vi "Preprocessor.vi"() -> ()   [LabVIEW 2018]
uses:
  <vilib>/userdefined/High Color/IMAQdx.ctl
  <vilib>/vision/driver/IMAQdx.llb/IMAQdx Buffer Number Mode.ctl
  <vilib>/vision/driver/NI_Vision_Acquisition_Software.lvlib
  <vilib>/vision/NI_Vision_Development_Module.lvlib
panel:
  out "Processed 3":T1(plugin-control)
  out "MulFLAG":i32
  out "FLAG":i32
  out "FLAG":u8
  in  "Stop":bool
  in  "选项卡控件":T2(tab)
  in  "Method Select":T3(tab)
  in  "Start":bool
  in  "BINARY RANGE":cluster{u8, u8}(slide) scale=0.255..255.0
  out "Histogram":T4(graph)
  in  "Show Histo":bool
  in  "Equalize":bool
  in  "Process":bool
  in  "Operator":T5(ring)
  in  "X Val":sgl
  in  "RGBorGrey":bool
  in  "Range":cluster{"Numeric":sgl, "Numeric":sgl}(slide) scale=0.0..255.0
  in  "PackorCanny":bool
  in  "CANNY":bool
  in  "EDGE":bool
  in  "Edge Pack":T6(ring)
  in  "Canny Params":T7
  in  "Enable":bool
  in  "LOW               HIGH":bool
  in  "Frequency":bool
  in  "Plane":T8(ring)
  in  "Truncation Frequency %":sgl=10.0 format="%.2f"
  in  "Default or Personal":bool
  in  "Enable 2":bool
  out "Array":sgl[][](array[numeric])
  in  "Kernel Size":i32=3 min=3 max=7 step=2
  in  "Method":T9(ring)
  in  "Enable 3":bool
  in  "Kernel":string
  in  "Select":u16(ring) items=["Processed", "Origin"]
  in  "Camera Setting":T10
  out "Origin":T1(plugin-control)
  out "Processed":T1(plugin-control)
  in  "Save Image":bool
  in  "File Path":path
  in  "File Name":string
  in  "Method Control":enum32{"Single Operation", "Multiple Operation"}(tab)
  in  "Grey Trans":bool
  in  "Blur":bool
  in  "Symmetry":bool
  in  "Shift":bool
  in  "Rotate":bool
  in  "Binary":bool
  in  "Grey Trans 2":bool
  in  "Enable":bool
  in  "Blur 2":bool
  in  "Symmetry 2":bool
  in  "Shift 2":bool
  in  "Rotate 2":bool
  in  "Binary 2":bool
  out "Loading...":i32(slide) scale=-1.0..16.0
  out "Output Data Directory Path":path
  in  "Choose File 2":bool
  in  "Image Name":string
  in  "Generate number":i32
  out "Source Data File Path":path
  in  "Image format":string(combo)
  in  "Choose File":bool
  out "Processed 2":T1(plugin-control)
  # "Display"
  # "- Processed -"
  # "- Origin -"
  # "Threshold Image Processing:\n\n1. Start to process.\n2. You can scale the bar to change the\nthreshold of the algorithm.\n3. Click the Save button to save the pr\nocessed image."
  # "Gray Transform:\n\n1. Click Start button.\n2. Change the operator.\n3. Equalize histogram.\n4. Click Save button to Save image."
  # "Grey"
  # "RGB"
  # "Edge Detection\n\n1. Click Detect button.\n2. Change the Edge Pack.\n3. You can also choose canny detector.\n4. Click Save button to Save image."
  # "Canny"
  # "Pack"
  # "Frequency Processing:\n\n1. Click To Frequency Domain button.\n2. Change the Plane, you'll see the fre-\nquency image after FFT and FFTshift.\n3. You can also filter image based on \nhigh pass filter or low pass filter.\n4. Click Save button to save processed\nimage."
  # "High pass and Low pass Filter"
  # "Frequency Processing:\n\n1. Choose Default Mode or Personal\nMode.\n2. Click Enable button.\n3. Save images if you want."
  # "Personal"
  # "Default"
  # "Source Data"
  # "- Image Preview -"
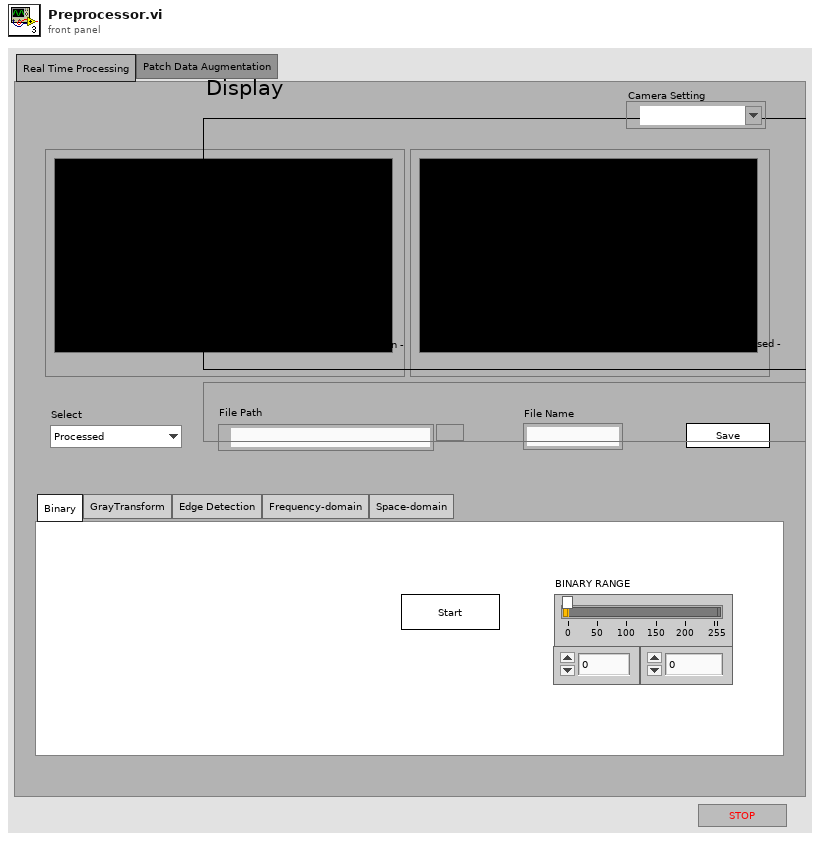
[diagram p1: front panel]
types:
  T1 = typedef "IMAQ Image.ctl" = refnum<image>
  T2 = enum32{"Real Time Processing", "Patch Data Augmentation"}
  T3 = enum32{"Binary", "GrayTransform", "Edge Detection", "Frequency-domain", "Space-domain"}
  T4 = cluster{"Starting Value":sgl, "Incremental Value":sgl, "Histogram":u32[]}
  T5 = enum32{"Linear", "Log", "Exp", "Square", "Square root", "Power X", "Power 1/X"}
  T6 = enum32{"Differentiation", "Gradient", "Prewitt", "Roberts", "Sigma", "Sobel"}
  T7 = cluster{"Sigma":sgl, "HThresh":sgl, "LThres":sgl, "WindowSize":i32}
  T8 = enum32{"Real", "Imaginary", "Magnitude", "Phase"}
  T9 = enum32{"", "Gradient", "Laplacian", "Smoothing", "Gaussian"}
  T10 = typedef "IMAQdx.ctl" = refnum<k21>
  T11 = typedef "Image Type" = u32
  T12 = typedef "NI_Vision_Acquisition_Software.lvlib/IMAQdx Buffer Number Mode.ctl" = enum32{"Next", "Last", "Buffer Number", "Every", "Last New"}
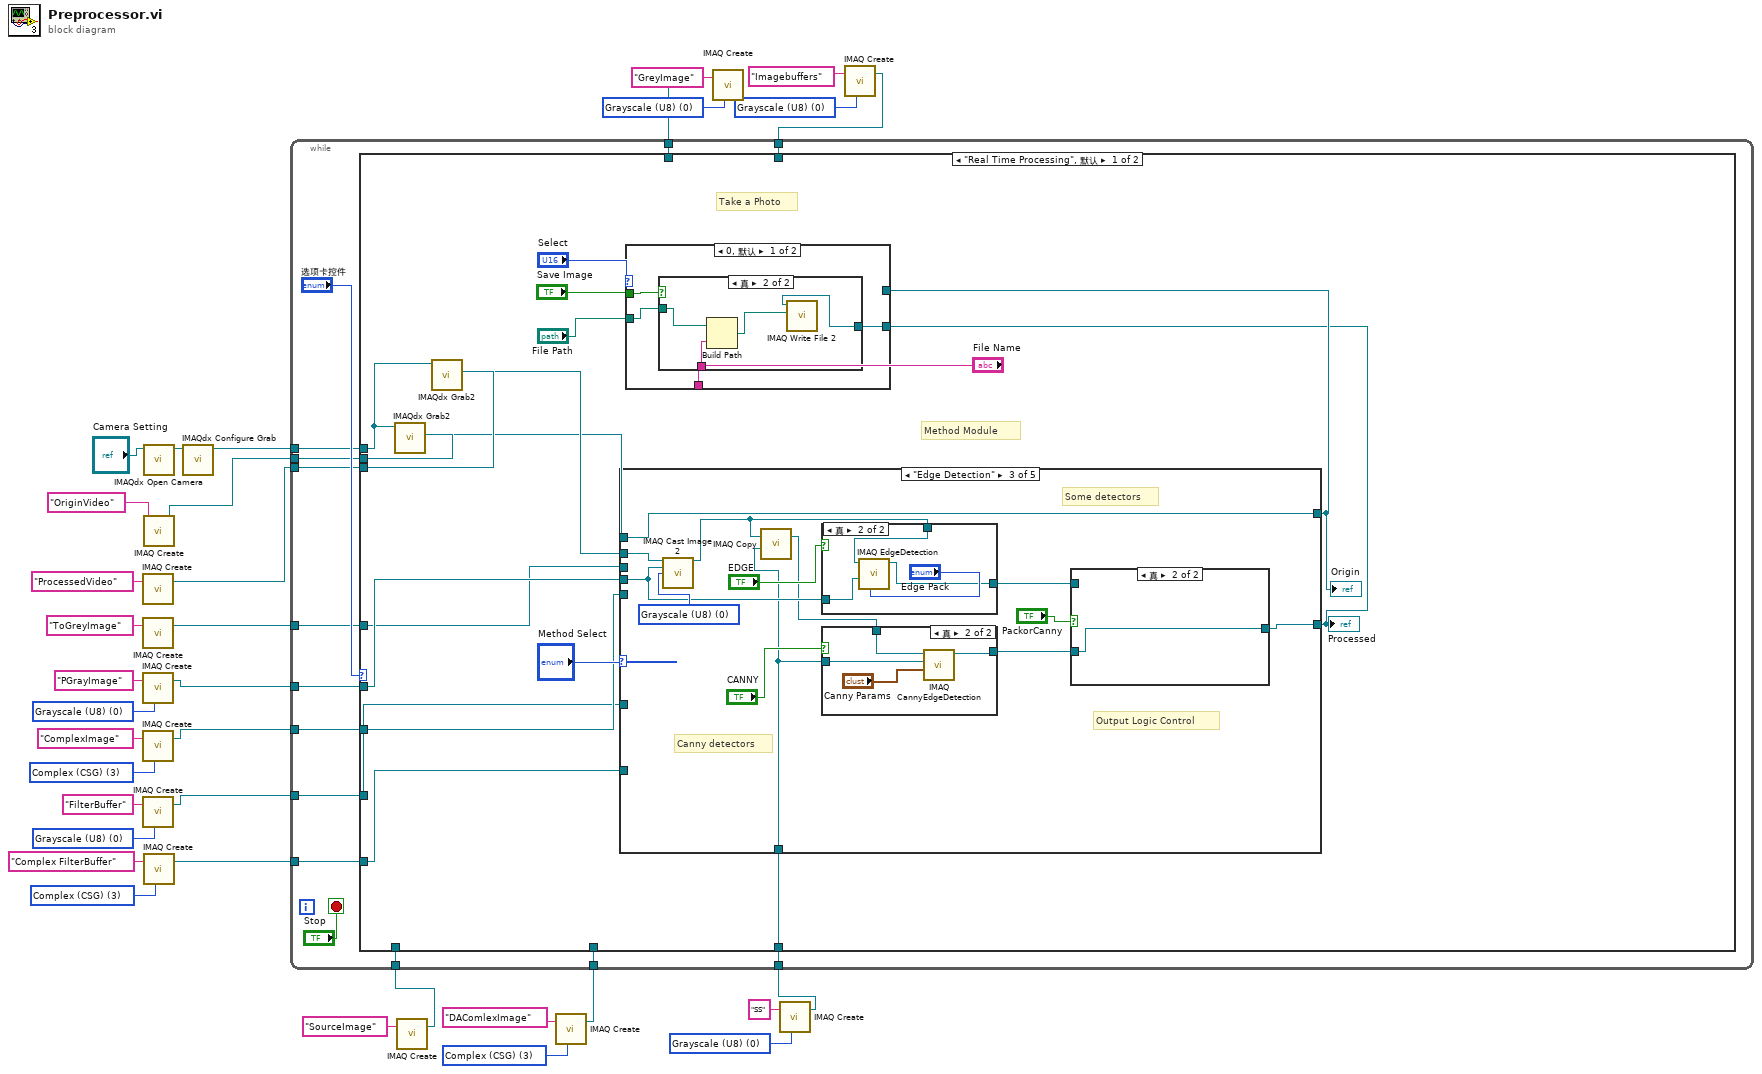
[diagram p0: block diagram]
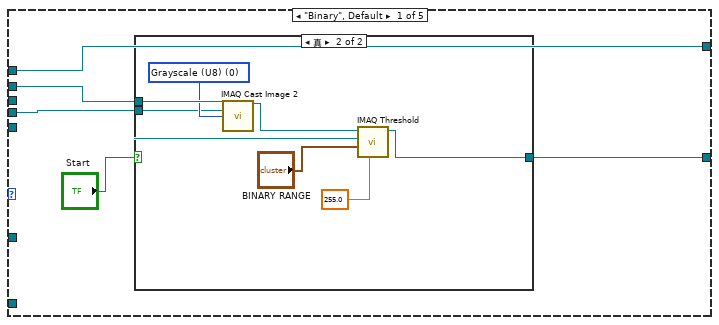
[diagram p2: hidden frame]
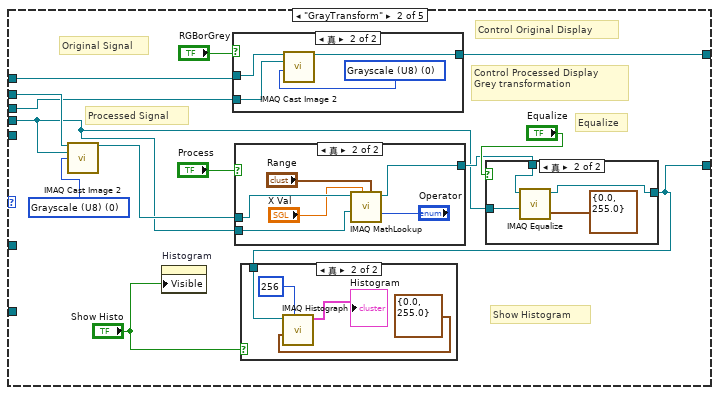
[diagram p4: hidden frame]
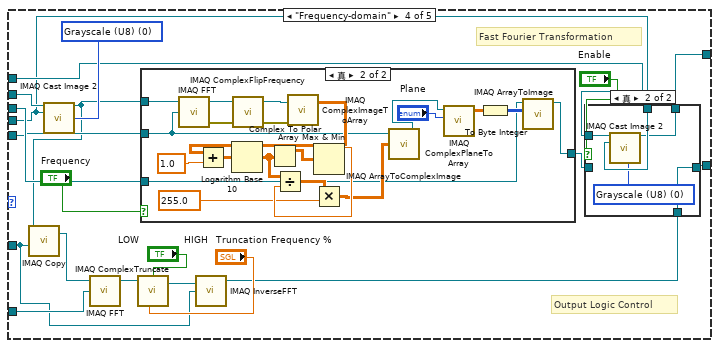
[diagram p12: hidden frame]
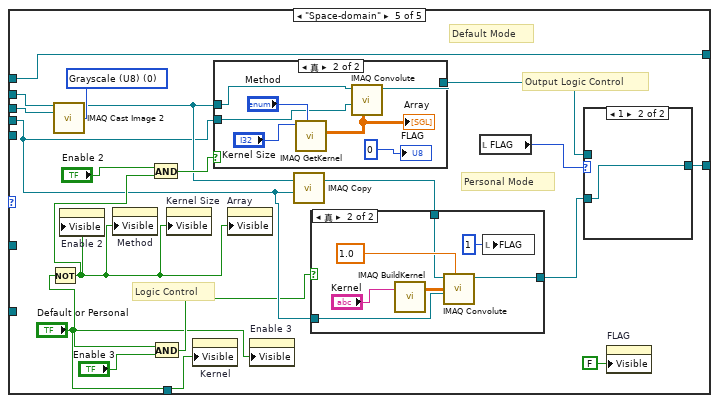
[diagram p15: hidden frame]
diagram:
  w3 = T11 0 items=["Grayscale (U8)", "Grayscale (I16)", "Grayscale (SGL)", "Complex (CSG)", "RGB (U32)", "HSL (U32)", "RGB (U64)", "Grayscale (U16)"] ("Image Type")
  w5 = T11 3 items=["Grayscale (U8)", "Grayscale (I16)", "Grayscale (SGL)", "Complex (CSG)", "RGB (U32)", "HSL (U32)", "RGB (U64)", "Grayscale (U16)"] ("Image Type")
  w8 = T11 0 items=["Grayscale (U8)", "Grayscale (I16)", "Grayscale (SGL)", "Complex (CSG)", "RGB (U32)", "HSL (U32)", "RGB (U64)", "Grayscale (U16)"] ("Image Type")
  w11 = T11 0 items=["Grayscale (U8)", "Grayscale (I16)", "Grayscale (SGL)", "Complex (CSG)", "RGB (U32)", "HSL (U32)", "RGB (U64)", "Grayscale (U16)"] ("Image Type")
  w16 = T11 3 items=["Grayscale (U8)", "Grayscale (I16)", "Grayscale (SGL)", "Complex (CSG)", "RGB (U32)", "HSL (U32)", "RGB (U64)", "Grayscale (U16)"] ("Image Type")
  w19 = T11 0 items=["Grayscale (U8)", "Grayscale (I16)", "Grayscale (SGL)", "Complex (CSG)", "RGB (U32)", "HSL (U32)", "RGB (U64)", "Grayscale (U16)"] ("Image Type")
  w22 = T11 3 items=["Grayscale (U8)", "Grayscale (I16)", "Grayscale (SGL)", "Complex (CSG)", "RGB (U32)", "HSL (U32)", "RGB (U64)", "Grayscale (U16)"] ("Image Type")
  w24 = T11 0 items=["Grayscale (U8)", "Grayscale (I16)", "Grayscale (SGL)", "Complex (CSG)", "RGB (U32)", "HSL (U32)", "RGB (U64)", "Grayscale (U16)"] ("Image Type")
  n1 = call "IMAQ Create"("Image Name"="ProcessedVideo") -> ("New Image"=w29:T1)  [unwired: 4 in, 1 out]
  n2 = call "IMAQ Create"("Image Name"="ToGreyImage") -> ("New Image"=w27:T1)  [unwired: 4 in, 1 out]
  n3 = call "IMAQ Create"("Image Name"="PGrayImage", "Image Type"=w24) -> ("New Image"=w25:T1)  [unwired: 3 in, 1 out]
  n4 = call "IMAQ Create"("Image Name"="ComplexImage", "Image Type"=w22) -> ("New Image"=w21:T1)  [unwired: 3 in, 1 out]
  n5 = call "IMAQ Create"("Image Name"="FilterBuffer", "Image Type"=w19) -> ("New Image"=w18:T1)  [unwired: 3 in, 1 out]
  n6 = call <vilib>:"IMAQdx Open Camera.vi"("Session In"="Camera Setting") -> ("Session Out"=w34:T10)  [unwired: 9 in, 1 out]
  n7 = call "IMAQ Create"("Image Name"="OriginVideo") -> ("New Image"=w31:T1)  [unwired: 4 in, 1 out]
  n8 = call "IMAQ Create"("Image Name"="Complex FilterBuffer", "Image Type"=w16) -> ("New Image"=w15:T1)  [unwired: 3 in, 1 out]
  n9 = call <vilib>:"IMAQdx Configure Grab.vi"("Session In"=w34) -> ("Session Out"=w32:T10)  [unwired: 9 in, 1 out]
  n10 = call "IMAQ Create"("Image Name"="SourceImage") -> ("New Image"=w13:T1)  [unwired: 4 in, 1 out]
  n11 = call "IMAQ Create"("Image Name"="DAComlexImage", "Image Type"=w5) -> ("New Image"=w4:T1)  [unwired: 3 in, 1 out]
  n12 = call "IMAQ Create"("Image Name"="GreyImage", "Image Type"=w11) -> ("New Image"=w10:T1)  [unwired: 3 in, 1 out]
  n13 = call "IMAQ Create"("Image Name"="SS", "Image Type"=w3) -> ("New Image"=w1:T1)  [unwired: 3 in, 1 out]
  n14 = call "IMAQ Create"("Image Name"="Imagebuffers", "Image Type"=w8) -> ("New Image"=w7:T1)  [unwired: 3 in, 1 out]
  n15 = while {
    tunnel: w32 -> [w48]
    tunnel: w31 -> [w47]
    tunnel: w29 -> [w46]
    tunnel: w27 -> [w45]
    tunnel: w25 -> [w44]
    tunnel: w21 -> [w43]
    tunnel: w18 -> [w42]
    tunnel: w15 -> [w41]
    tunnel: w13 -> [w40]
    tunnel: w10 -> [w39]
    tunnel: w7 -> [w38]
    tunnel: w4 -> [w37]
    tunnel: w1 -> [w36]
    stop <- "Stop" stop-if-true
    n16 = case shown="\"Real Time Processing\", 默认" "选项卡控件" {
      tunnel: w48 -> [w59 _]
      tunnel: w47 -> [w68 _]
      tunnel: w46 -> [w66 _]
      tunnel: w45 -> [w57 _]
      tunnel: w44 -> [w61 _]
      tunnel: w43 -> [w54 _]
      tunnel: w42 -> [w53 _]
      tunnel: w41 -> [w52 _]
      tunnel: w40 -> [_ w269]
      tunnel: w39 -> [_ w267]
      tunnel: w38 -> [_ w249]
      tunnel: w37 -> [_ w245]
      tunnel: w36 -> [w51 _]
      frame "Real Time Processing", Default {
        # "Take a Photo"
        # "Method Module"
        n17 = call <vilib>:"IMAQdx Grab2.vi"("Image In"=w68, "Session In"=w59) -> ("Image Out"=w58:T1)  [unwired: 6 in, 3 out]
        n18 = call <vilib>:"IMAQdx Grab2.vi"("Image In"=w66, "Session In"=w59) -> ("Image Out"=w60:T1)  [unwired: 6 in, 3 out]
        n19 = case shown="\"Edge Detection\"" "Method Select" {
          tunnel: w61 -> [w72 w84 w118 w142 w198]
          tunnel: w60 -> [w73 w94 w127 w160 w206]
          tunnel: w58 -> [w70 w91 w128 w143 w207]
          tunnel: [w70 w90 w128 w141 w207] -> w56
          tunnel: w57 -> [_ w89 _ w159 w205]
          tunnel: [w69 w83 w121 w151 w192] -> w55
          tunnel: w54 -> [_ _ _ w156 _]
          tunnel: w53 -> [_ _ _ w145 _]
          tunnel: w52 -> [_ _ _ w148 _]
          tunnel: w51 -> [_ _ w116 _ _]
          frame "Binary", Default {
            n20 = case shown="真" "Start" {
              tunnel: w73 -> [w74 w81]
              tunnel: w72 -> [_ w76]
              tunnel: [w74 w75] -> w69
              frame False {
              }
              frame True {
                w80 = T11 0 items=["Grayscale (U8)", "Grayscale (I16)", "Grayscale (SGL)", "Complex (CSG)", "RGB (U32)", "HSL (U32)", "RGB (U64)", "Grayscale (U16)"] ("Image Type")
                n21 = call "IMAQ Cast Image 2"("Image Src"=w81, "Image Dst"=w76, "Image Type"=w80) -> ("Image Dst Out"=w77:T1)  [unwired: 11 in, 1 out]
                n22 = call "IMAQ Threshold"("Replace Value"=sgl 255.0, "Range"="BINARY RANGE", "Image Dst"=w76, "Image Src"=w77) -> ("Image Dst Out"=w75:T1)  [unwired: 6 in, 1 out]
              }
            }
          }
          frame "GrayTransform" {
            w93 = T11 0 items=["Grayscale (U8)", "Grayscale (I16)", "Grayscale (SGL)", "Complex (CSG)", "RGB (U32)", "HSL (U32)", "RGB (U64)", "Grayscale (U16)"] ("Image Type")
            # "Show Histogram"
            # "Equalize"
            # "Processed Signal"
            # "Original Signal"
            # "Control Processed Display\nGrey transformation"
            # "Control Original Display"
            n23 = call "IMAQ Cast Image 2"("Image Src"=w94, "Image Dst"=w84, "Image Type"=w93) -> ("Image Dst Out"=w88:T1)  [unwired: 11 in, 1 out]
            n24 = property on="Histogram" class="WFGraph (严格)"("Visible"="Show Histo") -> ()  [unwired: 2 in, 2 out]
            n25 = case shown="真" "RGBorGrey" {
              tunnel: [w111 w113] -> w90
              tunnel: w91 -> [w111 w115]
              tunnel: w89 -> [_ w114]
              frame False {
              }
              frame True {
                w112 = T11 0 items=["Grayscale (U8)", "Grayscale (I16)", "Grayscale (SGL)", "Complex (CSG)", "RGB (U32)", "HSL (U32)", "RGB (U64)", "Grayscale (U16)"] ("Image Type")
                n26 = call "IMAQ Cast Image 2"("Image Src"=w115, "Image Dst"=w114, "Image Type"=w112) -> ("Image Dst Out"=w113:T1)  [unwired: 11 in, 1 out]
              }
            }
            n27 = case shown="真" "Process" {
              tunnel: w88 -> [w104 w108]
              tunnel: w84 -> [_ w106]
              tunnel: [w104 w105] -> w85
              frame False {
              }
              frame True {
                n28 = call "IMAQ MathLookup"("Range"="Range", "Operator"="Operator", "X Value"="X Val", "Image Dst"=w106, "Image Src"=w108) -> ("Image Dst Out"=w105:T1)  [unwired: 5 in, 1 out]
              }
            }
            n29 = case shown="真" "Equalize" {
              tunnel: w85 -> [w99 w102]
              tunnel: w84 -> [_ w101]
              tunnel: [w99 w100] -> w83
              frame False {
              }
              frame True {
                n30 = call "IMAQ Equalize"("Range"=cluster{"Minimum":sgl, "Maximum":sgl} {"Minimum"=0.0, "Maximum"=255.0} ("Interval Range"), "Image Dst"=w101, "Image Src"=w102) -> ("Image Dst Out"=w100:T1)  [unwired: 7 in, 1 out]
              }
            }
            n31 = case shown="真" "Show Histo" {
              tunnel: w83 -> [_ w95]
              frame False {
              }
              frame True {
                n32 = call "IMAQ Histograph"("Number of Classes"=256, "Interval Range"=cluster{"Minimum":sgl, "Maximum":sgl} {"Minimum"=0.0, "Maximum"=255.0}, "Image"=w95) -> ("Histogram Graph"=→"Histogram":T4)  [unwired: 5 in, 3 out]
              }
            }
          }
          frame "Edge Detection" {
            w126 = T11 0 items=["Grayscale (U8)", "Grayscale (I16)", "Grayscale (SGL)", "Complex (CSG)", "RGB (U32)", "HSL (U32)", "RGB (U64)", "Grayscale (U16)"] ("Image Type")
            # "Output Logic Control"
            # "Canny detectors"
            # "Some detectors"
            n33 = call "IMAQ Cast Image 2"("Image Src"=w127, "Image Dst"=w118, "Image Type"=w126) -> ("Image Dst Out"=w119:T1)  [unwired: 11 in, 1 out]
            n34 = call "IMAQ Copy"("Image Dst"=w116, "Image Src"=w119) -> ("Image Dst Out"=w117:T1)  [unwired: 4 in, 1 out]
            n35 = case shown="真" "EDGE" {
              tunnel: w119 -> [w136 w139]
              tunnel: w118 -> [_ w138]
              tunnel: [w136 w137] -> w122
              frame False {
              }
              frame True {
                n36 = call "IMAQ EdgeDetection"("Method"="Edge Pack", "Image Dst"=w138, "Image Src"=w139) -> ("Image Dst Out"=w137:T1)  [unwired: 7 in, 1 out]
              }
            }
            n37 = case shown="真" "CANNY" {
              tunnel: [w131 w134] -> w120
              tunnel: w117 -> [w131 w133]
              tunnel: w116 -> [_ w132]
              frame False {
              }
              frame True {
                n38 = call "IMAQ CannyEdgeDetection"("Image Src"=w133, "Image Dst"=w132, "Filter Parameters"="Canny Params") -> ("Image Dst Out"=w134:T1)  [unwired: 5 in, 1 out]
              }
            }
            n39 = case shown="真" "PackorCanny" {
              tunnel: [w129 w130] -> w121
              tunnel: w122 -> [w129 _]
              tunnel: w120 -> [_ w130]
              frame False {
              }
              frame True {
              }
            }
          }
          frame "Frequency-domain" {
            w158 = T11 0 items=["Grayscale (U8)", "Grayscale (I16)", "Grayscale (SGL)", "Complex (CSG)", "RGB (U32)", "HSL (U32)", "RGB (U64)", "Grayscale (U16)"] ("Image Type")
            # "Output Logic Control"
            # "Fast Fourier Transformation"
            n40 = call "IMAQ Cast Image 2"("Image Src"=w160, "Image Dst"=w142, "Image Type"=w158) -> ("Image Dst Out"=w150:T1)  [unwired: 11 in, 1 out]
            n41 = call "IMAQ Copy"("Image Dst"=w145, "Image Src"=w150) -> ("Image Dst Out"=w149:T1)  [unwired: 4 in, 1 out]
            n42 = call "IMAQ FFT"("Image Dst"=w148, "Image Src"=w149) -> ("Image Dst Out"=w147:T1)  [unwired: 2 in, 1 out]
            n43 = call "IMAQ ComplexTruncate"("Truncation Frequency %"="Truncation Frequency %", "Image Src"=w147, "Low pass/High pass (Low pass)"="LOW               HIGH") -> ("Image Dst Out"=w146:T1)  [unwired: 4 in, 1 out]
            n44 = case shown="真" "Frequency" {
              tunnel: w150 -> [w168 w173]
              tunnel: w159 -> [_ w172]
              tunnel: [w168 w171] -> w152
              tunnel: w156 -> [_ w170]
              frame False {
              }
              frame True {
                n45 = call "IMAQ FFT"("Image Dst"=w170, "Image Src"=w173) -> ("error out"=w187:errorcluster, "Image Dst Out"=w189:T1)  [unwired: 2 in]
                n46 = call "IMAQ ComplexFlipFrequency"("error in (no error)"=w187, "Image Src"=w189) -> ("error out"=w185:errorcluster, "Image Dst Out"=w186:T1)  [unwired: 2 in]
                n47 = call "IMAQ ComplexImageToArray"("Image"=w186, "error in (no error)"=w185) -> ("Image Pixels (Complex)"=w175:csg[][])  [unwired: 3 in, 1 out]
                n48 = Add(x=w175, y=1.0) -> (x+y=w177:cdb[][])
                n49 = Logarithm Base 10(1:w177) -> (0:w178:cdb[][])
                n50 = Complex To Polar(r * e^(i*theta)=w178) -> (r=w184:dbl[][])  [unwired: 1 out]
                n51 = Array Max & Min(array=w184) -> (max value=w183:dbl)  [unwired: 3 out]
                n52 = Divide(x=w178, y=w183) -> (x/y=w181:cdb[][])
                n53 = Multiply(x=w181, y=255.0) -> (x*y=w180:cdb[][])
                n54 = call "IMAQ ArrayToComplexImage"("Image Pixels (Complex)"=w180, "Image"=w170) -> ("Image Out"=w179:T1)  [unwired: 2 in, 1 out]
                n55 = call "IMAQ ComplexPlaneToArray"("Plane"="Plane", "Image"=w179) -> ("Image Pixels (float)"=w188:sgl[][])  [unwired: 3 in, 1 out]
                n56 = To Byte Integer(number=w188) -> (8bit integer=w174:i8[][])
                n57 = call "IMAQ ArrayToImage"("Image Pixels (U8)"=w174, "Image"=w172) -> ("Image Out"=w171:T1)  [unwired: 8 in, 1 out]
              }
            }
            n58 = call "IMAQ InverseFFT"("Image Dst"=w145, "Image Src"=w146) -> ("Image Dst Out"=w144:T1)  [unwired: 2 in, 1 out]
            n59 = case shown="真" "Enable" {
              tunnel: [w162 w167] -> w151
              tunnel: w152 -> [w162 _]
              tunnel: w144 -> [_ w167]
              tunnel: w143 -> [w161 w166]
              tunnel: w142 -> [_ w165]
              tunnel: [w161 w164] -> w141
              frame False {
              }
              frame True {
                w163 = T11 0 items=["Grayscale (U8)", "Grayscale (I16)", "Grayscale (SGL)", "Complex (CSG)", "RGB (U32)", "HSL (U32)", "RGB (U64)", "Grayscale (U16)"] ("Image Type")
                n60 = call "IMAQ Cast Image 2"("Image Src"=w166, "Image Dst"=w165, "Image Type"=w163) -> ("Image Dst Out"=w164:T1)  [unwired: 11 in, 1 out]
              }
            }
          }
          frame "Space-domain" {
            w204 = T11 0 items=["Grayscale (U8)", "Grayscale (I16)", "Grayscale (SGL)", "Complex (CSG)", "RGB (U32)", "HSL (U32)", "RGB (U64)", "Grayscale (U16)"] ("Image Type")
            # "Output Logic Control"
            # "Logic Control"
            # "Personal Mode"
            # "Default Mode"
            n61 = Not(x="Default or Personal") -> (.not. x?=w202:bool)
            n62 = call "IMAQ Cast Image 2"("Image Src"=w206, "Image Dst"=w205, "Image Type"=w204) -> ("Image Dst Out"=w200:T1)  [unwired: 11 in, 1 out]
            n63 = property on="Enable 2" class="Bool (严格)"("Visible"=w202) -> ()  [unwired: 2 in, 2 out]
            n64 = property on="Method" class="Enum (严格)"("Visible"=w202) -> ()  [unwired: 2 in, 2 out]
            n65 = And(x="Enable 2", y=w202) -> (x .and. y?=w201:bool)
            n66 = And(x="Default or Personal", y="Enable 3") -> (x .and. y?=w196:bool)
            n67 = property on="Kernel Size" class="DigNum (严格)"("Visible"=w202) -> ()  [unwired: 2 in, 2 out]
            n68 = property on="Kernel" class="Str"("Visible"="Default or Personal") -> ()  [unwired: 2 in, 2 out]
            n69 = case shown="真" w201 {
              tunnel: w200 -> [w218 w222]
              tunnel: w198 -> [_ w221]
              tunnel: [w218 w220] -> w193
              frame False {
              }
              frame True {
                n70 = call "IMAQ GetKernel"("Kernel Family"="Method", "Kernel Size (3,5,...)"="Kernel Size") -> ("Kernel"=w225:sgl[][])  [unwired: 6 in, 3 out]
                "Array" <- w225
                n71 = call "IMAQ Convolute"("Kernel"=w225, "Image Dst"=w221, "Image Src"=w222) -> ("Image Dst Out"=w220:T1)  [unwired: 7 in, 1 out]
                "FLAG" <- u8 0
              }
            }
            n72 = property on="Array" class="Arr (严格)"("Visible"=w202) -> ()  [unwired: 2 in, 2 out]
            n73 = property on="Enable 3" class="Bool (严格)"("Visible"="Default or Personal") -> ()  [unwired: 2 in, 2 out]
            n74 = call "IMAQ Copy"("Image Dst"=w198, "Image Src"=w200) -> ("Image Dst Out"=w199:T1)  [unwired: 4 in, 1 out]
            n75 = case shown="真" w196 {
              tunnel: w199 -> [_ w214]
              tunnel: w198 -> [w210 w213]
              tunnel: [w210 w211] -> w191
              frame False {
              }
              frame True {
                (unwired) 2 ("Window Number (0...15)")
                n76 = call "IMAQ BuildKernel"("Kernel String"="Kernel") -> ("Kernel"=w217:sgl[][])  [unwired: 4 in, 1 out]
                n77 = call "IMAQ Convolute"("Kernel"=w217, "Divider (kernel sum)"=sgl 1.0, "Image Dst"=w213, "Image Src"=w214) -> ("Image Dst Out"=w211:T1)  [unwired: 6 in, 1 out]
                n78 = local write "FLAG"(u8 1 ("数值")) -> ()
              }
            }
            n79 = local read "FLAG"() -> (w194:u8)
            n80 = case shown="1" w194 {
              tunnel: w193 -> [w208 _]
              tunnel: [w208 w209] -> w192
              tunnel: w191 -> [_ w209]
              frame 0, Default {
              }
              frame 1 {
              }
            }
            n81 = property on="FLAG" class="DigNum (严格)"("Visible"=FALSE ("可见")) -> ()  [unwired: 2 in, 2 out]
          }
        }
        "Processed" <- w55
        "Origin" <- w56
        n82 = case shown="0, 默认" "Select" {
          tunnel: "Save Image" -> [w229 w237]
          tunnel: "File Path" -> [w228 w236]
          tunnel: "File Name" -> [w227 w235]
          tunnel: w56 -> [_ w234]
          tunnel: w55 -> [w226 _]
          frame 0, Default {
            n83 = case shown="真" w229 {
              tunnel: w228 -> [_ w232]
              tunnel: w227 -> [_ w231]
              tunnel: w226 -> [_ w230]
              frame False {
              }
              frame True {
                n84 = Build Path(base path=w232, name or relative path=w231) -> (appended path=w233:path)
                n85 = call-poly "IMAQ Write File 2"("File Path"=w233, "Image"=w230) -> ()  [unwired: 8 in, 2 out]
              }
            }
          }
          frame 1 {
            n86 = case shown="假" w237 {
              tunnel: w236 -> [_ w240]
              tunnel: w235 -> [_ w239]
              tunnel: w234 -> [_ w238]
              frame False {
              }
              frame True {
                (unwired) IMAQdx_Buffer_Number_Mode."Last" ("Buffer Number Mode (Next)")
                n87 = Build Path(base path=w240, name or relative path=w239) -> (appended path=w241:path)
                n88 = call-poly "IMAQ Write File 2"("File Path"=w241, "Image"=w238) -> ()  [unwired: 8 in, 2 out]
              }
            }
          }
        }
      }
      frame "Patch Data Augmentation" {
        w242 = FALSE
        w266 = T11 0 items=["Grayscale (U8)", "Grayscale (I16)", "Grayscale (SGL)", "Complex (CSG)", "RGB (U32)", "HSL (U32)", "RGB (U64)", "Grayscale (U16)"] ("Image Type")
        # "Multiple Operation"
        # "Single Operation"
        # "Sate Register"
        # "Source File Path"
        # "Save Path"
        # "Button Group"
        # "Dst"
        # "Source"
        n89 = local read "FLAG"() -> (w262:i32)
        n90 = case shown="真" "Choose File" {
          tunnel: w269 -> [w557 w560]
          tunnel: [w557 w559] -> w268
          frame False {
          }
          frame True {
            n91 = call "File Dialog"() -> ("selected path"=w558:path)  [unwired: 12 in, 3 out]
            "Source Data File Path" <- w558
            n92 = call "IMAQ ReadFile 2"("File Path"=w558, "Image"=w560) -> ("Image Out"=w559:T1)  [unwired: 5 in, 4 out]
            "Processed 2" <- w559
          }
        }
        n93 = property on="Loading..." class="Slide (严格)"("Scale.Maximum"="Generate number") -> ()  [unwired: 2 in, 2 out]
        n94 = call "IMAQ Cast Image 2"("Image Src"=w268, "Image Dst"=w267, "Image Type"=w266) -> ("Image Dst Out"=w250:T1)  [unwired: 11 in, 1 out]
        n95 = case shown="6" w262 {
          tunnel: w250 -> [_ w402 w423 w449 w474 w498 w526]
          tunnel: w249 -> [_ w401 w422 w448 w473 w496 w525]
          tunnel: "Generate number" -> [_ w400 w424 w450 w475 w499 w524]
          tunnel: w245 -> [_ _ _ _ _ w497 _]
          frame 0, Default {
          }
          frame 1 {
            n96 = flat-sequence {
              tunnel: w402 -> [w405]
              tunnel: w401 -> [w404]
              tunnel: w400 -> [w403]
              frame #0 {
                n97 = for {
                  N: w403 -> [_]
                  tunnel: w405 -> [w420]
                  tunnel: w404 -> [w419]
                  i -> [w414]
                  n98 = local read "Image Name"() -> (w413:string)
                  n99 = Random Number (0-1)() -> (number: 0 to 1=w418:dbl)
                  n100 = Increment(x=w414) -> (x+1=w415:i32)
                  n101 = Multiply(x=w418, y=360.0) -> (x*y=w416:dbl)
                  n102 = Number To Decimal String(number=w414) -> (decimal integer string=w412:string)  [unwired: 1 in]
                  n103 = local write "Loading..."(w415) -> ()
                  n104 = local read "Image format"() -> (w410:string)
                  n105 = Concatenate Strings(w413, w412) -> (w411:string)
                  n106 = call "IMAQ Rotate"("Angle (degrees)"=w416, "Image Dst"=w419, "Image Src"=w420) -> ("Image Dst Out"=w406:T1)  [unwired: 7 in, 1 out]
                  n107 = local read "Output Data Directory Path"() -> (w409:path)
                  n108 = Concatenate Strings(w411, w410) -> (w408:string)
                  n109 = Build Path(base path=w409, name or relative path=w408) -> (appended path=w407:path)
                  n110 = call-poly "IMAQ Write File 2"("File Path"=w407, "Image"=w406) -> ()  [unwired: 8 in, 2 out]
                }
              }
              frame #1 {
                n111 = local write "FLAG"(0 ("FLAG")) -> ()
              }
            }
          }
          frame 2 {
            n112 = flat-sequence {
              tunnel: w424 -> [w427]
              tunnel: w423 -> [w426]
              tunnel: w422 -> [w425]
              frame #0 {
                n113 = for {
                  N: w427 -> [_]
                  tunnel: w426 -> [w432]
                  tunnel: w425 -> [w431]
                  i -> [w428]
                  n114 = Random Number (0-1)() -> (number: 0 to 1=w443:dbl)
                  n115 = Increment(x=w428) -> (x+1=→"Loading...":i32)
                  n116 = Multiply(x=w443, y=255.0) -> (x*y=w444:dbl)
                  n117 = Build Array(0.0, w444) -> (w445:dbl[])
                  n118 = Array To Cluster(array=w445) -> (cluster=w446:cluster{"[0]":dbl, "[1]":dbl})
                  n119 = call "IMAQ Threshold"("Replace Value"=sgl 255.0, "Range"=w446, "Image Dst"=w431, "Image Src"=w432) -> ("Image Dst Out"=w433:T1)  [unwired: 6 in, 1 out]
                  n120 = Number To Decimal String(number=w428) -> (decimal integer string=w437:string)  [unwired: 1 in]
                  n121 = local read "Output Data Directory Path"() -> (w430:path)
                  n122 = Concatenate Strings("Image Name", w437) -> (w436:string)
                  n123 = Concatenate Strings(w436, "Image format") -> (w435:string)
                  n124 = Build Path(base path=w430, name or relative path=w435) -> (appended path=w434:path)
                  n125 = call-poly "IMAQ Write File 2"("File Path"=w434, "Image"=w433) -> ()  [unwired: 8 in, 2 out]
                }
              }
              frame #1 {
                n126 = local write "FLAG"(0 ("数值")) -> ()
              }
            }
          }
          frame 3 {
            n127 = flat-sequence {
              tunnel: w450 -> [w453]
              tunnel: w449 -> [w452]
              tunnel: w448 -> [w451]
              frame #0 {
                n128 = for {
                  N: w453 -> [_]
                  tunnel: w452 -> [w471]
                  tunnel: w451 -> [w470]
                  i -> [w462]
                  n129 = Random Number (0-1)() -> (number: 0 to 1=w468:dbl)
                  n130 = Random Number (0-1)() -> (number: 0 to 1=w466:dbl)
                  n131 = local read "Image Name"() -> (w460:string)
                  n132 = Multiply(x=w468, y=200.0) -> (x*y=w467:dbl)
                  n133 = Multiply(x=w466, y=300.0) -> (x*y=w464:dbl)
                  n134 = Increment(x=w462) -> (x+1=w463:i32)
                  n135 = local read "Image format"() -> (w459:string)
                  n136 = Number To Decimal String(number=w462) -> (decimal integer string=w461:string)  [unwired: 1 in]
                  n137 = local write "Loading..."(w463) -> ()
                  n138 = Concatenate Strings(w460, w461) -> (w458:string)
                  n139 = local read "Output Data Directory Path"() -> (w455:path)
                  n140 = call "IMAQ Shift"("YOffset"=w464, "XOffset"=w467, "Image Dst"=w470, "Image Src"=w471) -> ("Image Dst Out"=w456:T1)  [unwired: 6 in, 1 out]
                  n141 = Concatenate Strings(w458, w459) -> (w457:string)
                  n142 = Build Path(base path=w455, name or relative path=w457) -> (appended path=w454:path)
                  n143 = call-poly "IMAQ Write File 2"("File Path"=w454, "Image"=w456) -> ()  [unwired: 8 in, 2 out]
                }
              }
              frame #1 {
                n144 = local write "FLAG"(0 ("FLAG")) -> ()
              }
            }
          }
          frame 4 {
            n145 = flat-sequence {
              tunnel: w475 -> [w478]
              tunnel: w474 -> [w477]
              tunnel: w473 -> [w476]
              frame #0 {
                n146 = for {
                  N: w478 -> [_]
                  tunnel: w477 -> [w483]
                  tunnel: w476 -> [w482]
                  i -> [w489]
                  n147 = local read "Image Name"() -> (w488:string)
                  n148 = Random Number (0-1)() -> (number: 0 to 1=w494:dbl)
                  n149 = local read "Image format"() -> (w480:string)
                  n150 = Increment(x=w489) -> (x+1=w490:i32)
                  n151 = Number To Decimal String(number=w489) -> (decimal integer string=w487:string)  [unwired: 1 in]
                  n152 = Multiply(x=w494, y=2) -> (x*y=w492:dbl)
                  n153 = local write "Loading..."(w490) -> ()
                  n154 = Round To Nearest(number=w492) -> (nearest integer value=w491:dbl)
                  n155 = Concatenate Strings(w488, w487) -> (w479:string)
                  n156 = Concatenate Strings(w479, w480) -> (w486:string)
                  n157 = local read "Output Data Directory Path"() -> (w485:path)
                  n158 = call "IMAQ Symmetry"("Type of Symmetry"=w491, "Image Dst"=w482, "Image Src"=w483) -> ("Image Dst Out"=w481:T1)  [unwired: 2 in, 1 out]
                  n159 = Build Path(base path=w485, name or relative path=w486) -> (appended path=w484:path)
                  n160 = call-poly "IMAQ Write File 2"("File Path"=w484, "Image"=w481) -> ()  [unwired: 8 in, 2 out]
                }
              }
              frame #1 {
                n161 = local write "FLAG"(0 ("FLAG")) -> ()
              }
            }
          }
          frame 5 {
            n162 = flat-sequence {
              tunnel: w499 -> [w503]
              tunnel: w498 -> [w502]
              tunnel: w497 -> [w501]
              tunnel: w496 -> [w500]
              frame #0 {
                n163 = for {
                  N: w503 -> [_]
                  tunnel: w502 -> [w513]
                  tunnel: w501 -> [w512]
                  tunnel: w500 -> [w509]
                  i -> [w521]
                  n164 = Random Number (0-1)() -> (number: 0 to 1=w507:dbl)
                  n165 = local read "Image Name"() -> (w520:string)
                  n166 = Increment(x=w521) -> (x+1=w522:i32)
                  n167 = Number To Decimal String(number=w521) -> (decimal integer string=w519:string)  [unwired: 1 in]
                  n168 = Multiply(x=w507, y=15.0) -> (x*y=w505:dbl)
                  n169 = local read "Image format"() -> (w518:string)
                  n170 = local write "Loading..."(w522) -> ()
                  n171 = call "IMAQ FFT"("Image Dst"=w512, "Image Src"=w513) -> ("Image Dst Out"=w511:T1)  [unwired: 2 in, 1 out]
                  n172 = Concatenate Strings(w520, w519) -> (w517:string)
                  n173 = call "IMAQ ComplexTruncate"("Truncation Frequency %"=w505, "Image Src"=w511, "Low pass/High pass (Low pass)"=FALSE) -> ("Image Dst Out"=w510:T1)  [unwired: 4 in, 1 out]
                  n174 = local read "Output Data Directory Path"() -> (w516:path)
                  n175 = Concatenate Strings(w517, w518) -> (w515:string)
                  n176 = call "IMAQ InverseFFT"("Image Dst"=w509, "Image Src"=w510) -> ("Image Dst Out"=w508:T1)  [unwired: 2 in, 1 out]
                  n177 = Build Path(base path=w516, name or relative path=w515) -> (appended path=w514:path)
                  n178 = call-poly "IMAQ Write File 2"("File Path"=w514, "Image"=w508) -> ()  [unwired: 8 in, 2 out]
                }
              }
              frame #1 {
                n179 = local write "FLAG"(0 ("FLAG")) -> ()
              }
            }
          }
          frame 6 {
            n180 = flat-sequence {
              tunnel: w526 -> [w529]
              tunnel: w525 -> [w528]
              tunnel: w524 -> [w527]
              frame #0 {
                n181 = for {
                  N: w527 -> [_]
                  tunnel: w529 -> [w541]
                  tunnel: w528 -> [w540]
                  i -> [w538]
                  n182 = local read "Image Name"() -> (w537:string)
                  n183 = Random Number (0-1)() -> (number: 0 to 1=w552:dbl)
                  n184 = Increment(x=w538) -> (x+1=w539:i32)
                  n185 = Multiply(x=w552, y=4) -> (x*y=w550:dbl)
                  n186 = Number To Decimal String(number=w538) -> (decimal integer string=w536:string)  [unwired: 1 in]
                  n187 = Round To Nearest(number=w550) -> (nearest integer value=w549:dbl)
                  n188 = local read "Image format"() -> (w535:string)
                  n189 = local write "Loading..."(w539) -> ()
                  n190 = Concatenate Strings(w537, w536) -> (w534:string)
                  n191 = Random Number (0-1)() -> (number: 0 to 1=w546:dbl)
                  n192 = Concatenate Strings(w534, w535) -> (w533:string)
                  n193 = local read "Output Data Directory Path"() -> (w532:path)
                  n194 = Multiply(x=w546, y=255.0) -> (x*y=w547:dbl)
                  n195 = Build Path(base path=w532, name or relative path=w533) -> (appended path=w531:path)
                  n196 = Build Array(0.0, w547) -> (w543:dbl[])
                  n197 = Array To Cluster(array=w543) -> (cluster=w542:cluster{"[0]":dbl, "[1]":dbl})
                  n198 = call "IMAQ MathLookup"("Range"=w542, "Operator"=w549, "X Value"=sgl 0.0, "Image Dst"=w540, "Image Src"=w541) -> ("Image Dst Out"=w530:T1)  [unwired: 5 in, 1 out]
                  n199 = call-poly "IMAQ Write File 2"("File Path"=w531, "Image"=w530) -> ()  [unwired: 8 in, 2 out]
                }
              }
              frame #1 {
                n200 = local write "FLAG"(0 ("FLAG")) -> ()
              }
            }
          }
        }
        n201 = case shown="真" "Choose File 2" {
          frame False {
          }
          frame True {
            n202 = call "文件对话框"() -> ("selected path"=→"Output Data Directory Path":path)  [unwired: 12 in, 3 out]
          }
        }
        n203 = property on="FLAG" class="DigNum (严格)"("Visible"=w242) -> ()  [unwired: 2 in, 2 out]
        n204 = property on="MulFLAG" class="DigNum (严格)"("Visible"=w242) -> ()  [unwired: 2 in, 2 out]
        n205 = local read "MulFLAG"() -> (w247:i32)
        n206 = property on="Processed 3" class="ImageControl"("Visible"=w242) -> ()  [unwired: 2 in, 2 out]
        n207 = case shown="真" "Binary" {
          frame False {
          }
          frame True {
            n208 = local write "FLAG"(2 ("数值")) -> ()
          }
        }
        n209 = Build Array("Binary 2", "Rotate 2", "Shift 2", "Symmetry 2", "Blur 2", "Grey Trans 2") -> (w251:bool[])
        n210 = case shown="1" w247 {
          tunnel: w251 -> [_ w276]
          tunnel: w250 -> [_ w275]
          tunnel: w249 -> [_ w274]
          tunnel: "Generate number" -> [_ w273]
          tunnel: w245 -> [_ w272]
          frame 0, Default {
          }
          frame 1 {
            n211 = flat-sequence {
              tunnel: w276 -> [w281]
              tunnel: w275 -> [w280]
              tunnel: w274 -> [w279]
              tunnel: w273 -> [w278]
              tunnel: w272 -> [w277]
              frame #0 {
                n212 = for {
                  N: w278 -> [_]
                  tunnel: w281 -> [w287]
                  tunnel: w280 -> [w283]
                  tunnel: w279 -> [w286]
                  tunnel: w277 -> [w282]
                  i -> [w284]
                  n213 = stacked-sequence {
                    tunnel: w287 -> [w292 w307 w320 w336 w351 w367 _]
                    tunnel: w286 -> [w289 w305 w318 w334 w348 w365 _]
                    tunnel: w284 -> [_ _ _ _ _ _ w387]
                    tunnel: w282 -> [_ _ _ _ w349 _ _]
                    frame #0 {
                      n214 = Boolean Array To Number(Boolean array=w292) -> (number=w294:u32)
                      n215 = And(x=w294, y=u32 1) -> (x .and. y?=w288:u32)
                      n216 = Equal?(x=w288, y=u32 1) -> (x = y?=w290:bool)
                      n217 = case shown="真" w290 {
                        tunnel: w289 -> [_ w297]
                        frame False {
                        }
                        frame True {
                          n218 = Random Number (0-1)() -> (number: 0 to 1=w303:dbl)
                          n219 = Multiply(x=w303, y=255.0) -> (x*y=w304:dbl)
                          n220 = Build Array(0.0, w304) -> (w300:dbl[])
                          n221 = Array To Cluster(array=w300) -> (cluster=w298:cluster{"[0]":dbl, "[1]":dbl})
                          n222 = local read "Processed 3"() -> (w296:T1)
                          n223 = call "IMAQ Threshold"("Replace Value"=sgl 255.0, "Range"=w298, "Image Dst"=w297, "Image Src"=w296) -> ("Image Dst Out"=w295:T1)  [unwired: 6 in, 1 out]
                          n224 = local write "Processed 3"(w295) -> ()
                        }
                      }
                    }
                    frame #1 {
                      n225 = Boolean Array To Number(Boolean array=w307) -> (number=w311:u32)
                      n226 = And(x=w311, y=u32 2) -> (x .and. y?=w309:u32)
                      n227 = Equal?(x=w309, y=u32 2) -> (x = y?=w306:bool)
                      n228 = case shown="真" w306 {
                        tunnel: w305 -> [_ w317]
                        frame False {
                        }
                        frame True {
                          n229 = Random Number (0-1)() -> (number: 0 to 1=w316:dbl)
                          n230 = Multiply(x=w316, y=360.0) -> (x*y=w314:dbl)
                          n231 = local read "Processed 3"() -> (w312:T1)
                          n232 = call "IMAQ Rotate"("Angle (degrees)"=w314, "Image Dst"=w317, "Image Src"=w312) -> ("Image Dst Out"=w313:T1)  [unwired: 7 in, 1 out]
                          n233 = local write "Processed 3"(w313) -> ()
                        }
                      }
                    }
                    frame #2 {
                      n234 = Boolean Array To Number(Boolean array=w320) -> (number=w324:u32)
                      n235 = And(x=w324, y=u32 4) -> (x .and. y?=w322:u32)
                      n236 = Equal?(x=w322, y=u32 4) -> (x = y?=w319:bool)
                      n237 = case shown="真" w319 {
                        tunnel: w318 -> [_ w325]
                        frame False {
                        }
                        frame True {
                          n238 = Random Number (0-1)() -> (number: 0 to 1=w331:dbl)
                          n239 = Random Number (0-1)() -> (number: 0 to 1=w332:dbl)
                          n240 = Multiply(x=w331, y=300.0) -> (x*y=w328:dbl)
                          n241 = Multiply(x=w332, y=200.0) -> (x*y=w329:dbl)
                          n242 = local read "Processed 3"() -> (w327:T1)
                          n243 = call "IMAQ Shift"("YOffset"=w328, "XOffset"=w329, "Image Dst"=w325, "Image Src"=w327) -> ("Image Dst Out"=w326:T1)  [unwired: 6 in, 1 out]
                          n244 = local write "Processed 3"(w326) -> ()
                        }
                      }
                    }
                    frame #3 {
                      n245 = Boolean Array To Number(Boolean array=w336) -> (number=w340:u32)
                      n246 = And(x=w340, y=u32 8) -> (x .and. y?=w338:u32)
                      n247 = Equal?(x=w338, y=u32 8) -> (x = y?=w335:bool)
                      n248 = case shown="真" w335 {
                        tunnel: w334 -> [_ w341]
                        frame False {
                        }
                        frame True {
                          n249 = Random Number (0-1)() -> (number: 0 to 1=w347:dbl)
                          n250 = Multiply(x=w347, y=2) -> (x*y=w345:dbl)
                          n251 = Round To Nearest(number=w345) -> (nearest integer value=w344:dbl)
                          n252 = local read "Processed 3"() -> (w343:T1)
                          n253 = call "IMAQ Symmetry"("Type of Symmetry"=w344, "Image Dst"=w341, "Image Src"=w343) -> ("Image Dst Out"=w342:T1)  [unwired: 2 in, 1 out]
                          n254 = local write "Processed 3"(w342) -> ()
                        }
                      }
                    }
                    frame #4 {
                      n255 = Boolean Array To Number(Boolean array=w351) -> (number=w355:u32)
                      n256 = And(x=w355, y=u32 16) -> (x .and. y?=w353:u32)
                      n257 = Equal?(x=w353, y=u32 16) -> (x = y?=w350:bool)
                      n258 = case shown="真" w350 {
                        tunnel: w349 -> [_ w363]
                        tunnel: w348 -> [_ w356]
                        frame False {
                        }
                        frame True {
                          n259 = Random Number (0-1)() -> (number: 0 to 1=w361:dbl)
                          n260 = Multiply(x=w361, y=15.0) -> (x*y=w359:dbl)
                          n261 = local read "Processed 3"() -> (w362:T1)
                          n262 = call "IMAQ FFT"("Image Dst"=w363, "Image Src"=w362) -> ("Image Dst Out"=w358:T1)  [unwired: 2 in, 1 out]
                          n263 = call "IMAQ ComplexTruncate"("Truncation Frequency %"=w359, "Image Src"=w358) -> ("Image Dst Out"=w357:T1)  [unwired: 5 in, 1 out]
                          n264 = call "IMAQ InverseFFT"("Image Dst"=w356, "Image Src"=w357) -> ("Image Dst Out"=w364:T1)  [unwired: 2 in, 1 out]
                          n265 = local write "Processed 3"(w364) -> ()
                        }
                      }
                    }
                    frame #5 {
                      n266 = Boolean Array To Number(Boolean array=w367) -> (number=w371:u32)
                      n267 = And(x=w371, y=u32 32) -> (x .and. y?=w369:u32)
                      n268 = Equal?(x=w369, y=u32 32) -> (x = y?=w366:bool)
                      n269 = case shown="真" w366 {
                        tunnel: w365 -> [_ w372]
                        frame False {
                        }
                        frame True {
                          n270 = Random Number (0-1)() -> (number: 0 to 1=w385:dbl)
                          n271 = local read "Processed 3"() -> (w373:T1)
                          n272 = Multiply(x=w385, y=4) -> (x*y=w383:dbl)
                          n273 = Round To Nearest(number=w383) -> (nearest integer value=w376:dbl)
                          n274 = Random Number (0-1)() -> (number: 0 to 1=w381:dbl)
                          n275 = Multiply(x=w381, y=255.0) -> (x*y=w382:dbl)
                          n276 = Build Array(0.0, w382) -> (w378:dbl[])
                          n277 = Array To Cluster(array=w378) -> (cluster=w375:cluster{"[0]":dbl, "[1]":dbl})
                          n278 = call "IMAQ MathLookup"("Range"=w375, "Operator"=w376, "X Value"=sgl 0.0, "Image Dst"=w372, "Image Src"=w373) -> ("Image Dst Out"=w374:T1)  [unwired: 5 in, 1 out]
                          n279 = local write "Processed 3"(w374) -> ()
                        }
                      }
                    }
                    frame #6 {
                      n280 = local read "Image Name"() -> (w388:string)
                      n281 = local read "Image format"() -> (w390:string)
                      n282 = Number To Decimal String(number=w387) -> (decimal integer string=w389:string)  [unwired: 1 in]
                      n283 = Concatenate Strings(w388, w389) -> (w391:string)
                      n284 = local read "Output Data Directory Path"() -> (w392:path)
                      n285 = Concatenate Strings(w391, w390) -> (w393:string)
                      n286 = Build Path(base path=w392, name or relative path=w393) -> (appended path=w394:path)
                      n287 = local read "Processed 3"() -> (w386:T1)
                      n288 = call-poly "IMAQ Write File 2"("File Path"=w394, "Image"=w386) -> ()  [unwired: 8 in, 2 out]
                    }
                  }
                  n289 = Increment(x=w284) -> (x+1=w285:i32)
                  n290 = local write "Loading..."(w285) -> ()
                  "Processed 3" <- w283
                }
              }
              frame #1 {
                n291 = local write "MulFLAG"(0 ("MulFLAG")) -> ()
              }
            }
          }
        }
        n292 = case shown="真" "Rotate" {
          frame False {
          }
          frame True {
            n293 = local write "FLAG"(1 ("数值")) -> ()
          }
        }
        n294 = case shown="真" "Shift" {
          frame False {
          }
          frame True {
            n295 = local write "FLAG"(3 ("FLAG")) -> ()
          }
        }
        n296 = case shown="真" "Symmetry" {
          frame False {
          }
          frame True {
            n297 = local write "FLAG"(4 ("FLAG")) -> ()
          }
        }
        n298 = case shown="真" "Blur" {
          frame False {
          }
          frame True {
            n299 = local write "FLAG"(5 ("FLAG")) -> ()
          }
        }
        n300 = case shown="真" "Enable" {
          frame False {
          }
          frame True {
            n301 = local write "MulFLAG"(1 ("MulFLAG")) -> ()
          }
        }
        n302 = case shown="真" "Grey Trans" {
          frame False {
          }
          frame True {
            n303 = local write "FLAG"(6 ("FLAG")) -> ()
          }
        }
        "FLAG" <- 0
        "MulFLAG" <- 0
      }
    }
  }
